vi "Start and stop activity (subVi).vi"(2 "error in":errorcluster, 3 "Text Ring":u16(ring) items=["Filament off/Saving off", "Filament on/Saving off", "Filament on/Saving on"]) -> (0 "error out":errorcluster)   [LabVIEW 2016]
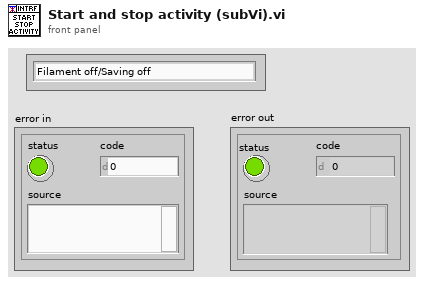
[diagram p1: front panel]
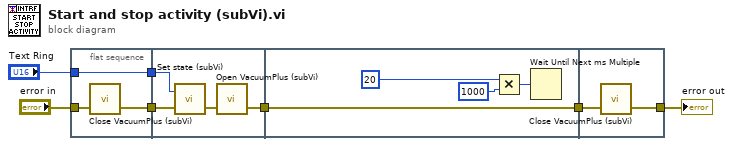
[diagram p0: block diagram]
diagram:
  n1 = flat-sequence {
    tunnel: "Text Ring" -> [w9]
    tunnel: "error in" -> [w10]
    tunnel: [w8] -> w2
    tunnel: [w9] -> w1
    tunnel: [w13] -> w7
    tunnel: w2 -> [w12]
    tunnel: w1 -> [w11]
    tunnel: w7 -> [w15]
    tunnel: [w15] -> w5
    tunnel: w5 -> [w20]
    tunnel: [w19] -> w4
    frame #0 {
      n2 = call "Close VacuumPlus (subVi).vi"("error in (no error)"=w10) -> ("error out"=w8:errorcluster)  [unwired: 1 in, 1 out]
    }
    frame #1 {
      n3 = call "Set state (subVi).vi"("error in"=w12, "Text Ring"=w11) -> ("error out"=w14:errorcluster)  [unwired: 1 in]
      n4 = call "Open VacuumPlus (subVi).vi"("error in (no error)"=w14) -> ("error out"=w13:errorcluster)  [unwired: 1 in, 1 out]
    }
    frame #2 {
      n5 = Multiply(x=20, y=1000) -> (x*y=w18:i32)
      n6 = Wait Until Next ms Multiple(millisecond multiple=w18) -> ()  [unwired: 1 out]
    }
    frame #3 {
      n7 = call "Close VacuumPlus (subVi).vi"("error in (no error)"=w20) -> ("error out"=w19:errorcluster)  [unwired: 1 in, 1 out]
    }
  }
  "error out" <- w4
